vi "generator.vi"(2 "Sygna³":T1(ring), 3 "Amplituda":dbl(knob) scale=0.0..10.0, 4 "Czêstotliwoœæ":dbl(knob) scale=0.0..10.0) -> (0 "Charakterystyka":waveform(dbl)(graph))   [LabVIEW 2020]
uses:
  <vilib>/measure/NI_MABase.lvlib
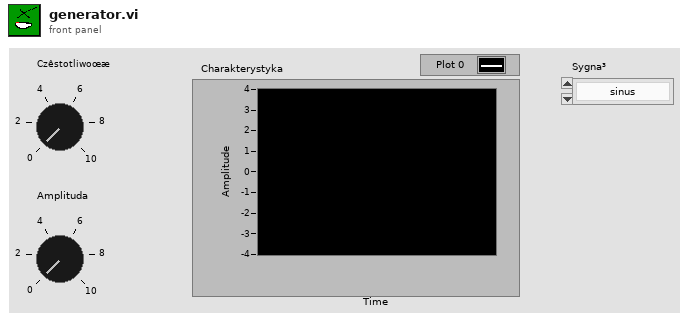
[diagram p1: front panel]
types:
  T1 = enum16{"sinus\n", "square\n", "triangle\n", "sawtooth\n"}
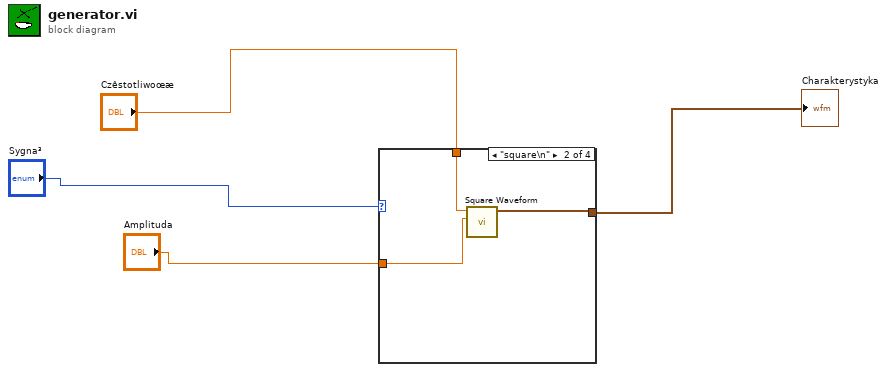
[diagram p0: block diagram]
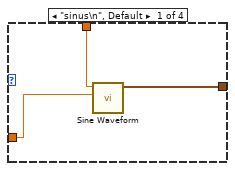
[diagram p2: hidden frame]
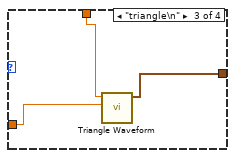
[diagram p3: hidden frame]
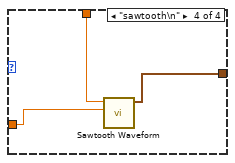
[diagram p4: hidden frame]
diagram:
  n1 = case shown="\"square\\n\"" "Sygna³" {
    tunnel: "Amplituda" -> [w7 w10 w13 w15]
    tunnel: "Czêstotliwoœæ" -> [w6 w9 w12 w16]
    tunnel: [w5 w8 w11 w14] -> w1
    frame "sinus\n", Default {
      n2 = call <vilib>:"Sine Waveform.vi"("amplitude"=w7, "frequency"=w6) -> ("signal out"=w5:waveform(dbl))  [unwired: 8 in, 1 out]
    }
    frame "square\n" {
      n3 = call <vilib>:"Square Waveform.vi"("amplitude"=w10, "frequency"=w9) -> ("signal out"=w8:waveform(dbl))  [unwired: 8 in, 1 out]
    }
    frame "triangle\n" {
      n4 = call <vilib>:"Triangle Waveform.vi"("amplitude"=w13, "frequency"=w12) -> ("signal out"=w11:waveform(dbl))  [unwired: 8 in, 1 out]
    }
    frame "sawtooth\n" {
      n5 = call <vilib>:"Sawtooth Waveform.vi"("amplitude"=w15, "frequency"=w16) -> ("signal out"=w14:waveform(dbl))  [unwired: 8 in, 1 out]
    }
  }
  "Charakterystyka" <- w1
